vi "Load Project.vi"(8 "error in (no error)":errorcluster, 11 "Edit Project Model in":refnum<class "Edit Project Model.lvclass">) -> (0 "error out":errorcluster, 3 "Edit Project Model out":refnum<class "Edit Project Model.lvclass">)   [LabVIEW 2013, in "Edit Project Model.lvlib" / "Edit Project Model.lvclass"]
uses:
  Edit Project Model.lvclass
  Edit Project Model.lvclass/Edit Project Model.ctl
  Common/File IO/File IO.lvlib
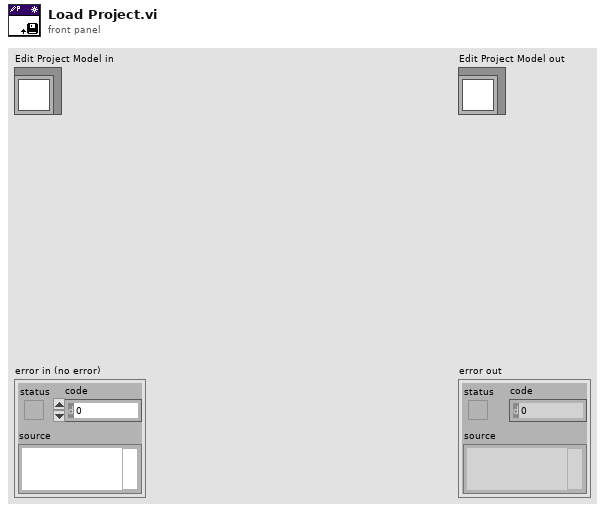
[diagram p1: front panel]
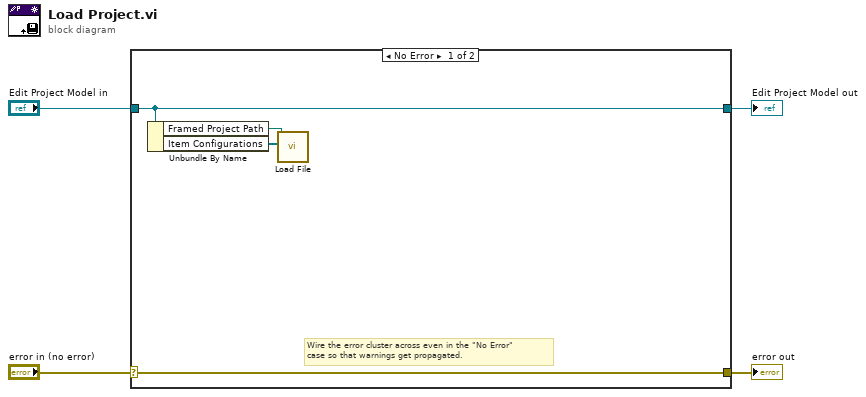
[diagram p0: block diagram]
diagram:
  n1 = case shown="No Error" "error in (no error)" {
    selector: "error in (no error)" -> [w8 w10]
    tunnel: [w8 w10] -> w3
    tunnel: [w7 w9] -> w1
    tunnel: "Edit Project Model in" -> [w7 w9]
    frame No Error {
      # "Wire the error cluster across even in the \"No Error\"\ncase so that warnings get propagated."
      n2 = Unbundle By Name(w7) -> ("Framed Project Path"=w6:path, "Item Configurations"=w5:refnum<class "Item Configuration.lvclass">[])
      n3 = call "Load File.vi"("Item Configurations"=w5, "File Path"=w6) -> ()  [unwired: 9 in, 1 out]
    }
    frame Error {
    }
  }
  "error out" <- w3
  "Edit Project Model out" <- w1
